vi "Pack AIP Command.vi"(11 "AIP Command":T1) -> (3 "AIP Deploy Command out":refnum<class "AIP Command.lvclass">)   [LabVIEW 2015, in "AIP Instrument.lvlib"]
uses:
  AIP Instrument.lvlib
  Libraries/RDS Framework/RDS Message Class/AIP Command Control.ctl
  Libraries/RDS Framework/RDS Message Class/AIP Command.lvclass
  Libraries/RDS Framework/RDS Message ID.ctl
  Libraries/RDS Framework/RDS Message Class/RDS Message.lvclass/RDS Message.ctl
  Libraries/RDS Framework/RDS Message Class/AIP Command.lvclass/AIP Command.ctl
  Libraries/RDS Framework/RDS Message Class/RDS Message.lvclass
  Libraries/RDS Child Messages/RDS Child Messages.lvlib
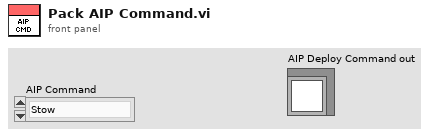
[diagram p1: front panel]
types:
  T1 = typedef "RDS Child Messages.lvlib/AIP Command Control.ctl" = enum16{"Stow", "Deploy", "Stop", "Validate Sensors", "Jog Deploy FP", "Jog Stow FP", "Jog Deploy FS", "Jog Stow FS", "Jog Deploy AP", "Jog Stow AP", "Jog Deploy AS", "Jog Stow AS", "Deploy FP", "Deploy FS", "Deploy AP", "Deploy AS", "Stow FP", "Stow FS", "Stow AP", "Stow AS"}
  T2 = typedef "RDS Child Messages.lvlib/RDS Message ID.ctl" = enum16{"RDS Hello World", "String Message", "AIP_Status", "AIP_Command", "GPS_Data", "MCB_Command", "MCB_Status", "Compass_Data", "Depth_Data", "Battery_Data", "Contoller_State", "Set_Mag_Dev", "BTB_Shutdown", "State_Sample_Request", "State_Sample", "PID_Gains_Set", "Helm_Limiter_Set", "Helm_Heading_Command", "Helm_Steering_Command", "Helm_Status", "Controller_Message", "AIP_Set_Min_Depth", "Mission_Controller_State", "Mission_Upload", "Mission_Set_Op_and_Run", "Mission_Settings_Set"}
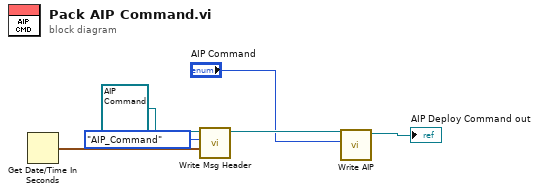
[diagram p0: block diagram]
diagram:
  n1 = Get Date/Time In Seconds() -> (seconds since 1Jan1904=w5:timestamp)
  n2 = call "Write Msg Header.vi"("Time Stamp"=w5, "Msg ID"=RDS_Message_ID."AIP_Command", "RDS Message in"=refnum<class "AIP Command.lvclass"> refnum ("RDS Child Messages.lvlib:AIP Command.lvclass")) -> ("RDS Message out"=w3:refnum<class "AIP Command.lvclass">)  [unwired: 7 in, 1 out]
  n3 = call "Write AIP.vi"("AIP Command"="AIP Command", "AIP Deploy Command in"=w3) -> ("AIP Deploy Command out"=→"AIP Deploy Command out":refnum<class "AIP Command.lvclass">)  [unwired: 8 in, 1 out]
